vi "WFPanel.vi"() -> ()   [LabVIEW 2012, in "StimulCtrls.lvlib"]
uses:
  StimulCtrls.lvlib
panel:
  out "Sequence 5":dbl(graph)
  in  "Stop Button":bool
  out "Sequence 4":dbl(graph)
  out "Sequence 3":dbl(graph)
  out "Sequence 2":dbl(graph)
  out "Sequence 1":dbl(graph)
  out "Sequence 0":dbl(graph)
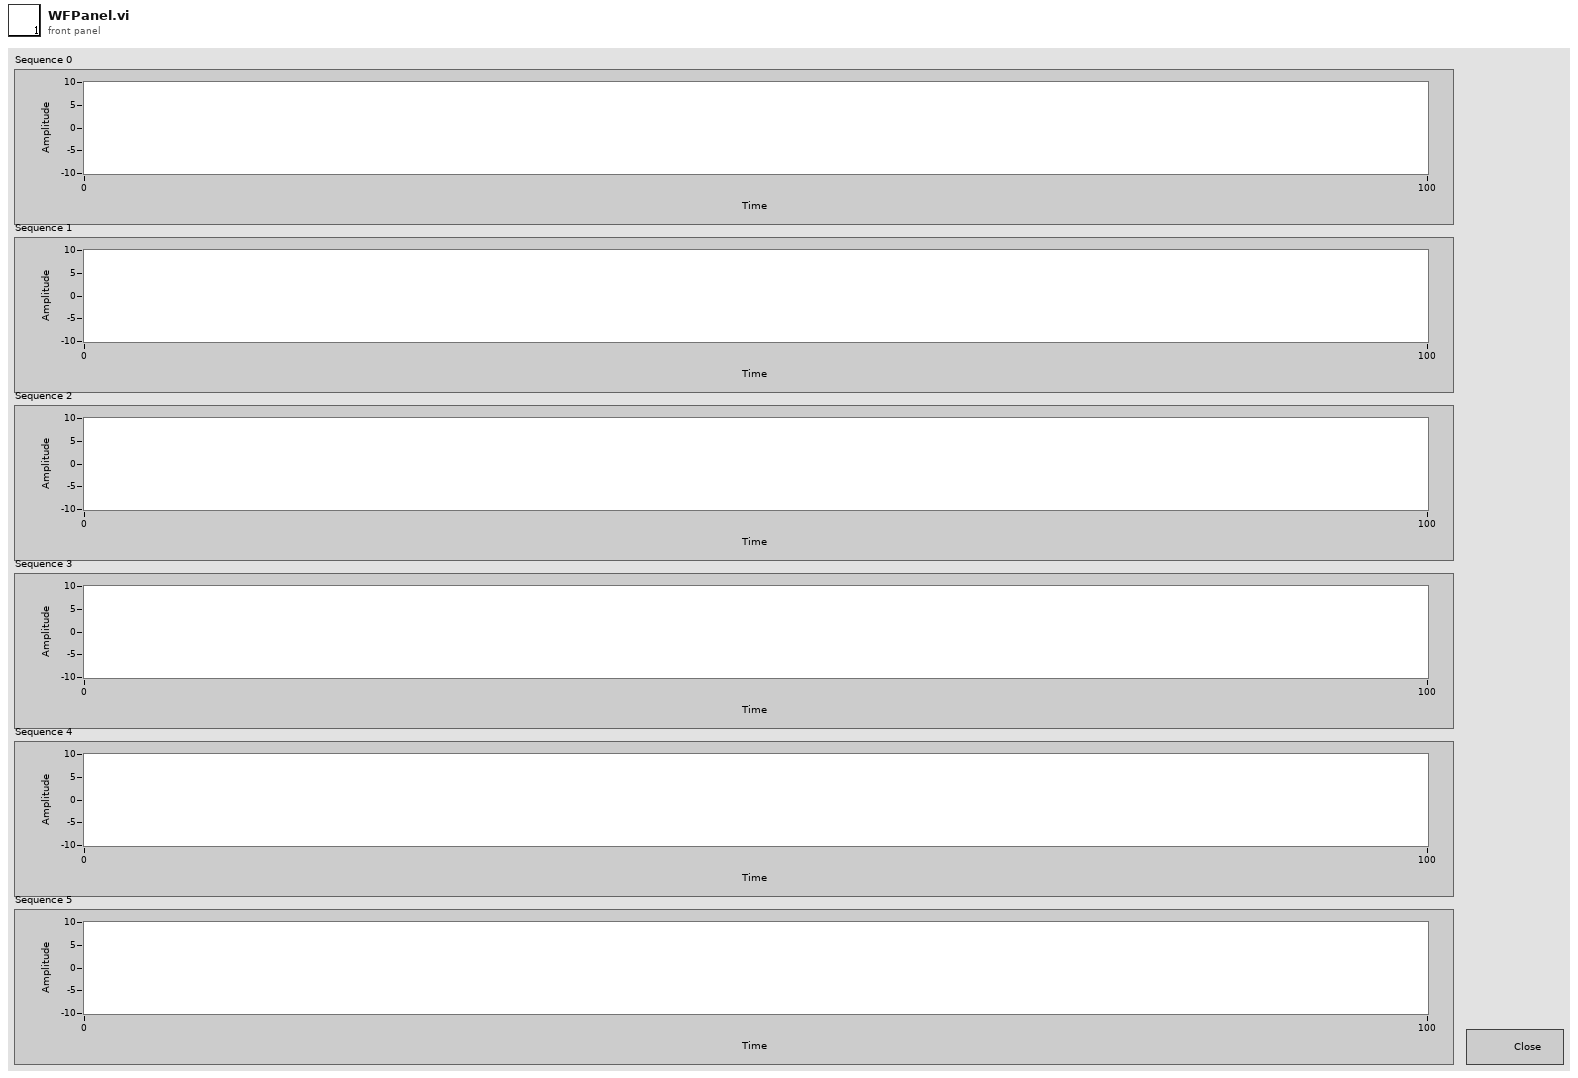
[diagram p1: front panel]
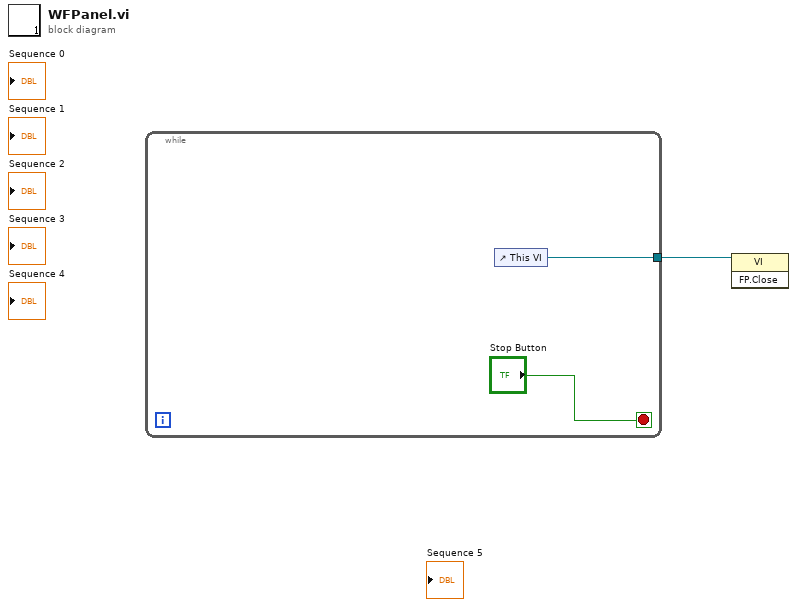
[diagram p0: block diagram]
diagram:
  n1 = while {
    tunnel: [w2] -> w1
    stop <- "Stop Button" stop-if-true
    n2 = control-ref of="This VI"() -> (w2:refnum<vi>)
  }
  n3 = invoke class="VI" method="FP.Close"(reference=w1) -> ()  [unwired: 2 in, 3 out]
